vi "Clear_RegDests.vi"(8 "error in (no error)":errorcluster, 11 "Class in":refnum<class "IB_MSI.lvclass">) -> (0 "error out":errorcluster, 3 "Class out":refnum<class "IB_MSI.lvclass">)   [LabVIEW 2020, in "IB_MSI.lvclass"]
uses:
  <vilib>/AppBuilder/IB_Classes/MSI/IB_MSI.lvclass
  <vilib>/AppBuilder/IB_Classes/MSI/IB_MSI.lvclass/IB_MSI.ctl
  <vilib>/AppBuilder/IB_Classes/Installer/Installer.lvclass
  <vilib>/AppBuilder/IB_Classes/RegDest/IB_RegDest.lvclass
  e:/builds/penguin/labview/branches/2020/dev/dist/vi.lib/AppBuilder/IB_Classes/Installer/Installer.lvclass
  e:/builds/penguin/labview/branches/2020/dev/dist/vi.lib/AppBuilder/IB_Classes/MSI/IB_MSI.lvclass
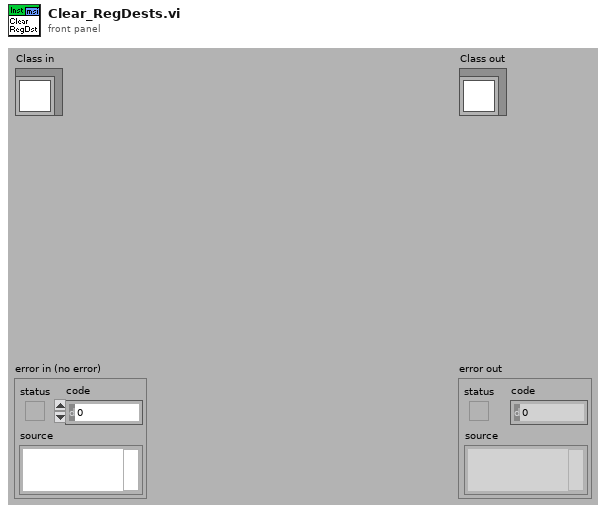
[diagram p1: front panel]
types:
  T1 = typedef "IB_Installer.ctl" = cluster{"Destination":refnum<class "IB_Destination.lvclass">[], "Source":refnum<class "IB_Source.lvclass">[], "buildObject":T2, "defaultDir":string, "platform":string, "author":string, "productName":string, "buildSpecName":string, "hide":bool, "requireLVDevSys":bool, "autoIncrement":bool, "includeError":bool, "readmeID":string, "buildLocation":path, "readmePath":path, "mediaSize":u16, "language":T3, "productVersion":T4, "preview":bool, "programmatic":bool, "progressBarEvents":T5, "userLog_Path":path, "shortcutAddresses":T7[], "EXE_Install Address":string, "EXE_Uninstall Address":string, "additional NIPaths":refnum<class "Dest_NI_NIPath.lvclass">[], "web service itemIDs":string[], "installerName":string}
  T2 = typedef "ItemRef.ctl" = u64
  T3 = typedef "CDK_sTypeDef_Languages.ctl" = u16
  T4 = typedef "CDK_sTypeDef_ProductVersion.ctl" = cluster{"Major":u8, "Minor":u8, "Update":u16}
  T5 = typedef "provcom_ProgressBar_Events.ctl" = cluster{"newJob":refnum<user-event>, "newItem":refnum<user-event>, "errorMsg":T6, "cancel":refnum<user-event>}
  T6 = typedef "mxLvBuildError.ctl" = refnum<user-event>
  T7 = typedef "CDK_sTypeDef_ShortcutAddress.ctl" = cluster{"file":string, "shortcut":string}
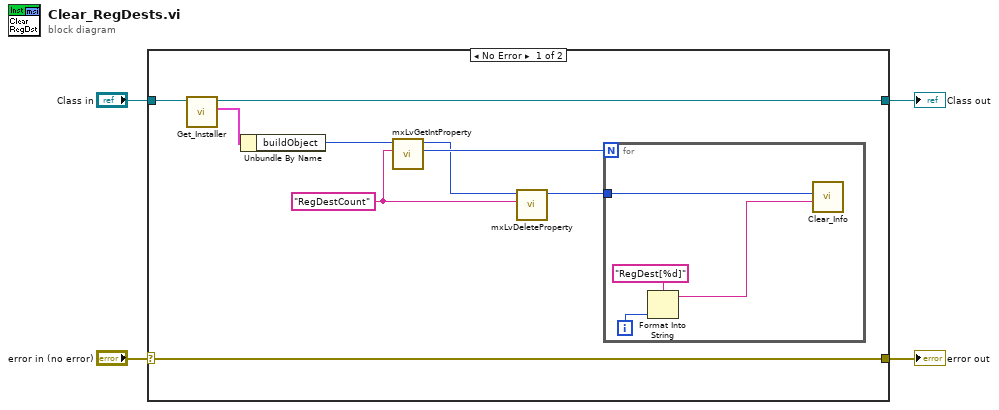
[diagram p0: block diagram]
diagram:
  n1 = case shown="No Error" "error in (no error)" {
    selector: "error in (no error)" -> [w11 w19]
    tunnel: [w11 w19] -> w3
    tunnel: [w10 w18] -> w1
    tunnel: "Class in" -> [w13 w18]
    frame No Error {
      w7 = "RegDestCount"
      n2 = call <vilib>:"Get_Installer.vi"("Installer in"=w13) -> ("data"=w12:T1, "Installer out"=w10:refnum<class "IB_MSI.lvclass">)  [unwired: 8 in, 1 out]
      n3 = Unbundle By Name(w12) -> ("buildObject"=w6:T2)
      n4 = call <resource>:"mxLvGetIntProperty.vi"("Tag"=w7, "Item"=w6) -> ("Value"=w8:i32, "Item"=w5:T2)  [unwired: 1 in, 7 out]
      n5 = call <resource>:"mxLvDeleteProperty.vi"("Tag"=w7, "Item"=w5) -> ("Item"=w9:T2)  [unwired: 1 in, 8 out]
      n6 = for {
        N: w8 -> [_]
        tunnel: w9 -> [w17]
        i -> [w15]
        n7 = Format Into String(format string="RegDest[%d]", w15) -> (resulting string=w14:string)  [unwired: 2 in, 1 out]
        n8 = call <vilib>:"Clear_Info.vi"("index in"=w14, "buildObject"=w17) -> ()  [unwired: 7 in, 3 out]
      }
    }
    frame Error {
    }
  }
  "error out" <- w3
  "Class out" <- w1
